vi "Shape Dialog.vi"(8 "error in (no error)":errorcluster, 10 "ShapeRef":refnum<data-value>, 11 "Editor Handler in":refnum<class "Image Editor Handler.lvclass">) -> (0 "error out":errorcluster, 3 "Editor Handler out":refnum<class "Image Editor Handler.lvclass">)   [LabVIEW 2017, in "LV Image Editor Framework.lvlib" / "Image Editor Handler.lvclass"]
uses:
  <vilib>/LIEF/Image Editor Handler/Image Editor Handler.lvclass
  <vilib>/LIEF/Forms/Shape/Shape.lvclass
  <vilib>/LIEF/Image Editor Handler/Image Editor Handler.lvclass/Image Editor Handler.ctl
  <vilib>/LIEF/Forms/Selection/Selection.lvclass
  <vilib>/LIEF/Forms/Selection/Selection.lvclass/Selection.ctl
  <vilib>/LIEF/Forms/Shape/Shape.lvclass/Shape.ctl
  <vilib>/LIEF/Forms/Selection/Read Selected Shape.vi
  <vilib>/LIEF/Forms/Shape/Read Color.vi
panel:
  out "Name":string
  out "Shape Type:":string
  out "Color:":u32(colorbox)
  out "Size:":string
  out "Position:":string
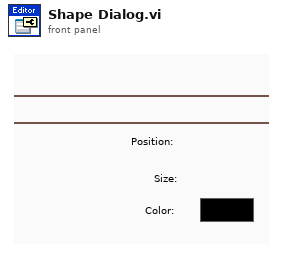
[diagram p1: front panel]
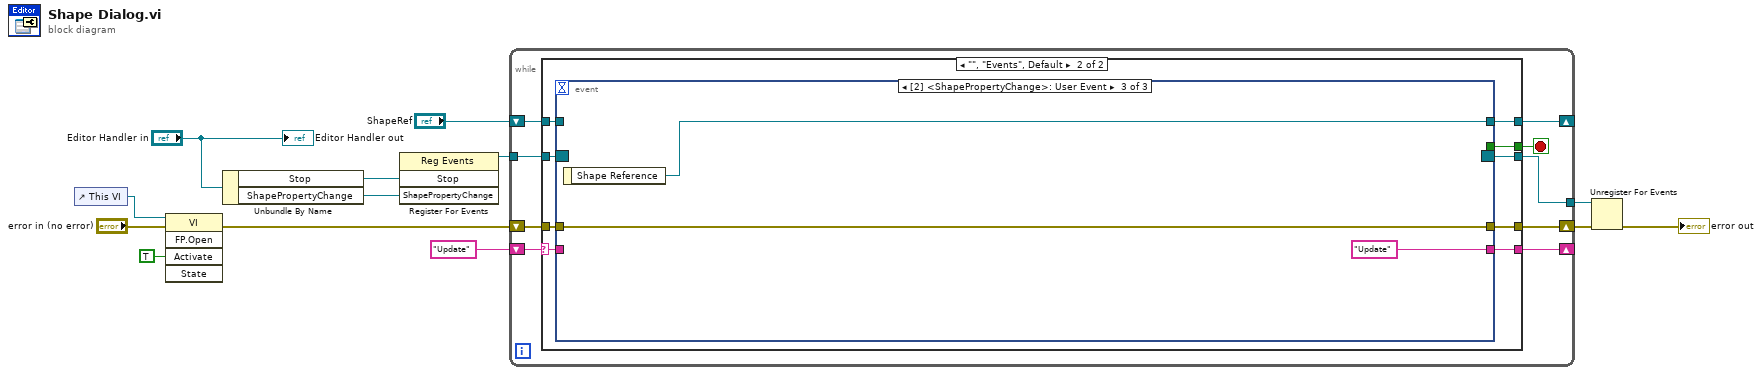
[diagram p0: block diagram]
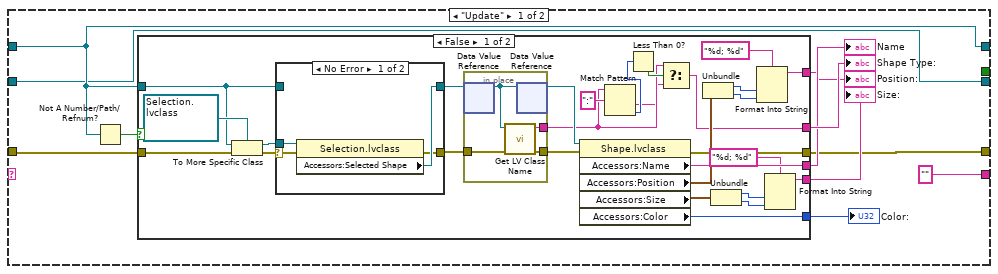
[diagram p2: hidden frame]
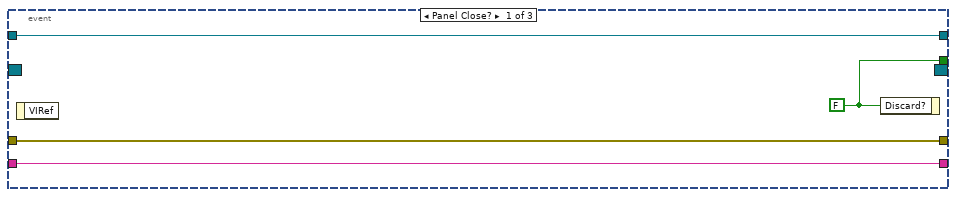
[diagram p5: hidden frame]
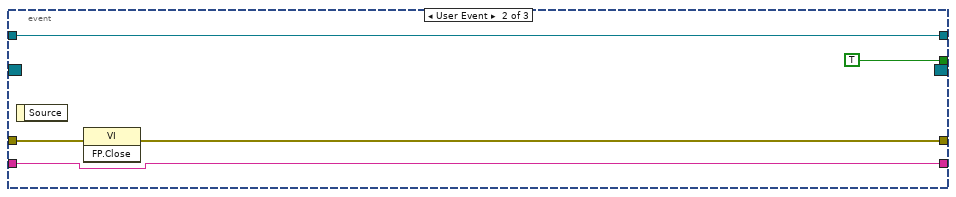
[diagram p6: hidden frame]
diagram:
  n1 = control-ref of="This VI"() -> (w12:refnum<vi>)
  n2 = invoke class="VI" method="FP.Open"(reference=w12, error in="error in (no error)", "Activate"=TRUE ("Activate?")) -> (error out=w5:errorcluster)  [unwired: 2 in, 4 out]
  n3 = Unbundle By Name("Editor Handler in") -> ("Stop"=w9:refnum<user-event>, "ShapePropertyChange"=w3:refnum<user-event>)
  n4 = register-events(w9, w3) -> (reference out=w8:refnum<event-registration>)  [unwired: 2 in, 1 out]
  n5 = while {
    shift-right: [w15] -> w6
    shift-left: w5 -> [w22]
    tunnel: w8 -> [w20]
    tunnel: [w19] -> w7
    shift-right: [w14] -> _
    shift-left: "Update" -> [w18]
    shift-right: [w17] -> _
    shift-left: "ShapeRef" -> [w16]
    stop <- w21 stop-if-true
    n6 = case shown="\"\", \"Events\", Default" w18 {
      selector: w18 -> [_ w72]
      tunnel: w22 -> [w27 w77]
      tunnel: [_ w80] -> w21
      tunnel: w20 -> [w25 w79]
      tunnel: [w25 w78] -> w19
      tunnel: [w26 w76] -> w17
      tunnel: w16 -> [w26 w75]
      tunnel: [w24 w74] -> w15
      tunnel: ["" w73] -> w14
      frame "Update" {
        n7 = Not A Number/Path/Refnum?(number/path/refnum=w26) -> (NaN/Path/Refnum?=w32:bool)
        n8 = case shown="False" w32 {
          tunnel: [w61 _] -> w33
          tunnel: [w60 _] -> w30
          tunnel: w27 -> [w54 w71]
          tunnel: [w53 w71] -> w24
          tunnel: [w34 _] -> w31
          tunnel: w26 -> [w50 _]
          tunnel: [w45 _] -> w29
          tunnel: [w40 _] -> w28
          frame False {
            n9 = To More Specific Class(target class=refnum<data-value> refnum ("Shape"), reference=w50, error in=w54) -> (specific class reference=w56:refnum<data-value>, error out=w55:errorcluster)
            n10 = case shown="No Error" w55 {
              selector: w55 -> [w68 _]
              tunnel: w56 -> [w69 _]
              tunnel: w50 -> [_ w70]
              tunnel: [w67 w70] -> w58
              tunnel: [w66 _] -> w51
              frame No Error {
                n11 = property class="Selection.lvclass"(reference=w69, error in=w68) -> (error out=w66:errorcluster, "Accessors:Selected Shape"=w67:refnum<data-value>)  [unwired: 1 out]
              }
              frame Error {
              }
            }
            n12 = in-place {
              in-place-border: [w65] -> w52
              in-place-border: w51 -> [w64]
              in-place-border: [w62] -> w36
              n13 = in-place-dvr #1(w58) -> (w63:refnum<class "Shape.lvclass">)  [unwired: 1 out]
              n14 = call <vilib>:"Get LV Class Name.vi"("error in (no error)"=w64, "object"=w63) -> ("error out"=w65:errorcluster, "class name"=w62:string)  [unwired: 8 in]
              n15 = in-place-dvr #1(w63) -> (w59:refnum<data-value>)  [unwired: 1 out]
            }
            n16 = property class="Shape.lvclass"(reference=w59, error in=w52) -> (error out=w53:errorcluster, "Accessors:Name"=w60:string, "Accessors:Position"=w48:cluster{"Left":i32, "Top":i32}, "Accessors:Size"=w41:cluster{"Width":i32, "Height":i32}, "Accessors:Color"=w61:u32)  [unwired: 1 out]
            n17 = Match Pattern(string=w36, regular expression=":") -> (after substring=w35:string, offset past match=w38:i32)  [unwired: 1 in, 2 out]
            n18 = Less Than 0?(x=w38) -> (x < 0?=w37:bool)
            n19 = Select(t=w36, s=w37, f=w35) -> (s? t:f=w34:string)
            n20 = Unbundle(w48) -> ("Left"=w49:i32, "Top"=w47:i32)
            n21 = Unbundle(w41) -> ("Width"=w43:i32, "Height"=w44:i32)
            n22 = Format Into String(format string="%d; %d", w49, w47) -> (resulting string=w45:string)  [unwired: 2 in, 1 out]
            n23 = Format Into String(format string="%d; %d", w43, w44) -> (resulting string=w40:string)  [unwired: 2 in, 1 out]
          }
          frame True {
          }
        }
        "Color:" <- w33
        "Position:" <- w29
        "Size:" <- w28
        "Shape Type:" <- w31
        "Name" <- w30
      }
      frame "", "Events", Default {
        n24 = event shown="[2] <ShapePropertyChange>: User Event" {
          selector: w79 -> [_ _ _]
          dyn-events: [_ _ _] -> w78
          timeout: _ -> [_ _ _]
          tunnel: w77 -> [w84 w88 w91]
          tunnel: [w84 w87 w91] -> w74
          tunnel: [w83 TRUE _] -> w80
          tunnel: [w82 w86 w92] -> w76
          tunnel: w75 -> [w82 w86 _]
          tunnel: [w81 w85 "Update"] -> w73
          tunnel: w72 -> [w81 w85 _]
          event Panel Close? {
            w83 = FALSE ("Discard?")
            n25 = event-data() -> ()  [unwired: 1 in, 1 out]
            n26 = event-data("Discard?"=w83) -> ()  [unwired: 1 in, 1 out]
          }
          event User Event {
            n27 = event-data() -> ()  [unwired: 1 in, 1 out]
            n28 = invoke class="VI" method="FP.Close"(error in=w88) -> (error out=w87:errorcluster)  [unwired: 2 in, 2 out]
          }
          event User Event {
            n29 = event-data() -> ("Shape Reference"=w92:refnum<data-value>)  [unwired: 1 in]
          }
        }
      }
    }
  }
  n30 = Unregister For Events(event registration refnum=w7, error in=w6) -> (error out=→"error out":errorcluster)
  "Editor Handler out" <- "Editor Handler in"
